vi "Load Drivers Dialog.vi"(8 "error in (no error)":errorcluster, 11 "Message Queue in":refnum<queue>) -> (0 "error out":errorcluster, 2 "Mssgs Sent":string, 5 "Asyncs":string[](array[string]), 7 "Syncs":string[](array[string]))   [LabVIEW 2014]
uses:
  APIs/Message Queue/Message Cluster.ctl
  APIs/Message Queue/Enqueue Message (Array).vi
  APIs/Message Queue/WINFAS 2 Message Queue.lvlib
panel:
  in  "LOAD":bool
  in  "Cancel":bool
  in  "Driver 5":path
  in  "Driver 4":path
  in  "Driver 3":path
  in  "Driver 2":path
  in  "Drivers Async":path[](array[path])=[path "", path "", path "", path "", path "", path "", path "", path "", path "", path ""]
  in  "Driver 1":path
  # "Drivers\nAsync"
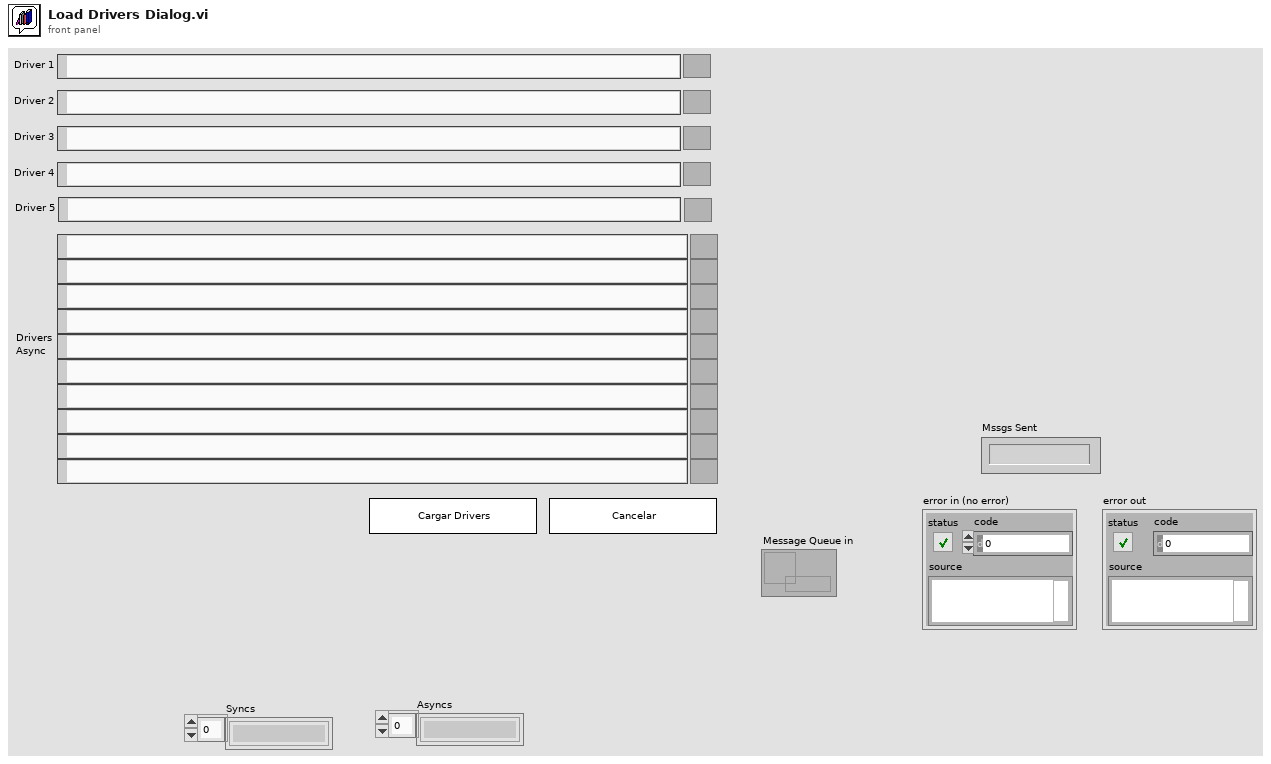
[diagram p1: front panel]
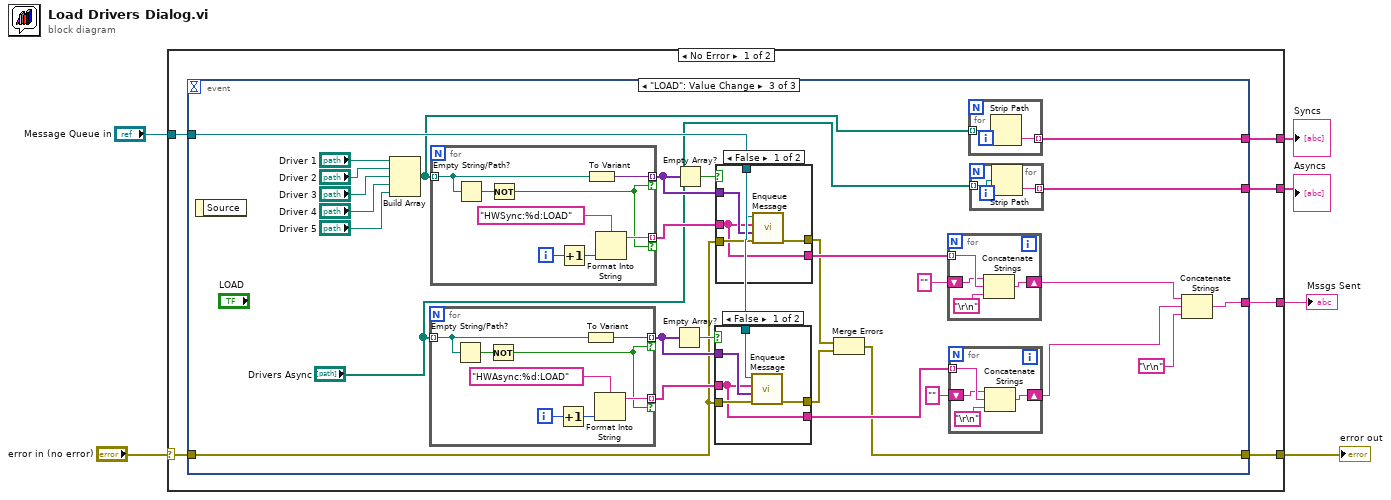
[diagram p0: block diagram]
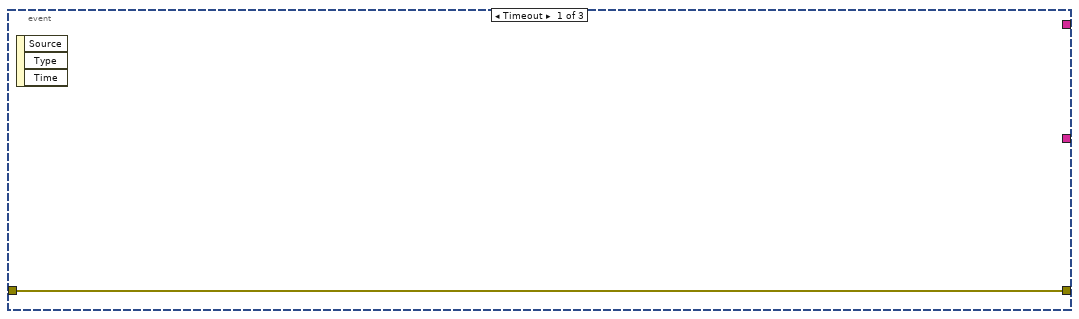
[diagram p2: hidden frame]
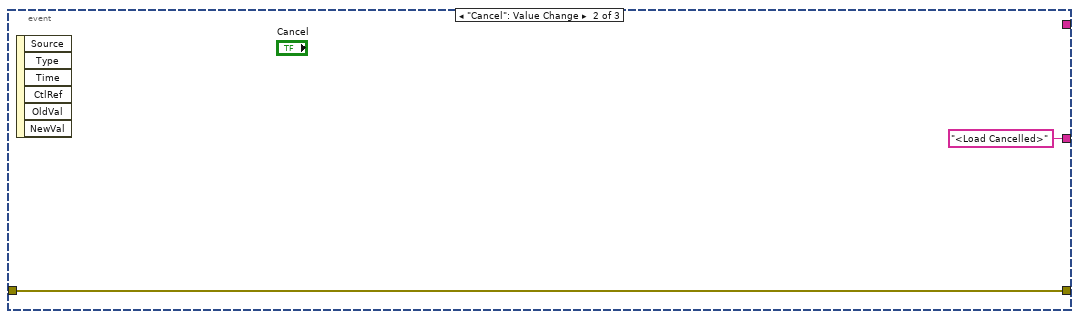
[diagram p3: hidden frame]
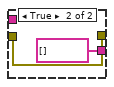
[diagram p4: hidden frame]
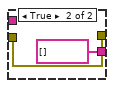
[diagram p5: hidden frame]
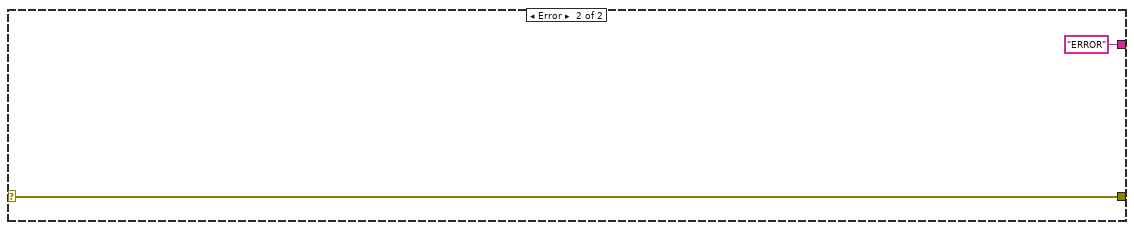
[diagram p6: hidden frame]
diagram:
  n1 = case shown="No Error" "error in (no error)" {
    selector: "error in (no error)" -> [w12 w87]
    tunnel: [w11 w87] -> w5
    tunnel: "Message Queue in" -> [w10 _]
    tunnel: [w9 "ERROR"] -> w3
    tunnel: [w8 _] -> w2
    tunnel: [w7 _] -> w1
    frame No Error {
      n2 = event shown="[2] \"LOAD\": Value Change" {
        selector: _ -> [_ _ _]
        dyn-events: _ -> [_ _ _]
        timeout: _ -> [_ _ _]
        tunnel: w12 -> [w13 w15 w20]
        tunnel: [w13 w15 w21] -> w11
        tunnel: w10 -> [_ _ w27]
        tunnel: [_ "<Load Cancelled>" w33] -> w9
        tunnel: [_ _ w17] -> w8
        tunnel: [_ _ w16] -> w7
        event Timeout {
          n3 = event-data() -> ()  [unwired: 1 in, 3 out]
        }
        event "Cancel": Value Change {
          n4 = event-data() -> ()  [unwired: 1 in, 6 out]
        }
        event "LOAD": Value Change {
          n5 = event-data() -> ()  [unwired: 1 in, 1 out]
          n6 = Build Array("Driver 1", "Driver 2", "Driver 3", "Driver 4", "Driver 5") -> (w19:path[])
          n7 = for {
            tunnel: "Drivers Async" -> [w62] mode=indexing
            tunnel: [w63] -> w29 mode=indexing if=w59
            tunnel: [w61] -> w30 mode=indexing if=w59
            i -> [w66]
            n8 = Empty String/Path?(string/path=w62) -> (empty?=w60:bool)
            n9 = Not(x=w60) -> (.not. x?=w59:bool)
            n10 = Increment(x=w66) -> (x+1=w64:i32)
            n11 = To Variant(anything=w62) -> (Variant=w61:variant)
            n12 = Format Into String(format string="HWAsync:%d:LOAD", w64) -> (resulting string=w63:string)  [unwired: 2 in, 1 out]
          }
          n13 = for {
            tunnel: w19 -> [w81] mode=indexing
            tunnel: [w82] -> w37 mode=indexing if=w78
            tunnel: [w80] -> w36 mode=indexing if=w78
            i -> [w85]
            n14 = Empty String/Path?(string/path=w81) -> (empty?=w79:bool)
            n15 = Not(x=w79) -> (.not. x?=w78:bool)
            n16 = Increment(x=w85) -> (x+1=w83:i32)
            n17 = To Variant(anything=w81) -> (Variant=w80:variant)
            n18 = Format Into String(format string="HWSync:%d:LOAD", w83) -> (resulting string=w82:string)  [unwired: 2 in, 1 out]
          }
          n19 = Empty Array?(array=w30) -> (empty?=w28:bool)
          n20 = Empty Array?(array=w36) -> (empty?=w38:bool)
          n21 = case shown="False" w28 {
            tunnel: [w56 w58] -> w22
            tunnel: w20 -> [w55 w58]
            tunnel: w27 -> [w54 _]
            tunnel: w29 -> [w52 _]
            tunnel: w30 -> [w53 _]
            tunnel: [w52 string[] []] -> w25
            frame False {
              n22 = call-poly "Enqueue Message.vi"("error in (no error)"=w55, "Message Data Array"=w53, "Message Array"=w52, "Message Queue"=w54) -> ("error out"=w56:errorcluster)  [unwired: 6 in, 1 out]
            }
            frame True {
            }
          }
          n23 = case shown="False" w38 {
            tunnel: [w75 w77] -> w23
            tunnel: w20 -> [w74 w77]
            tunnel: w27 -> [w73 _]
            tunnel: w37 -> [w71 _]
            tunnel: w36 -> [w72 _]
            tunnel: [w71 string[] []] -> w35
            frame False {
              n24 = call-poly "Enqueue Message.vi"("error in (no error)"=w74, "Message Data Array"=w72, "Message Array"=w71, "Message Queue"=w73) -> ("error out"=w75:errorcluster)  [unwired: 6 in, 1 out]
            }
            frame True {
            }
          }
          n25 = Merge Errors(w23, w22) -> (w21:errorcluster)
          n26 = for {
            tunnel: w35 -> [w70] mode=indexing
            shift-right: [w69] -> w34
            shift-left: "" -> [w68]
            n27 = Concatenate Strings(w68, w70, "\r\n") -> (w69:string)
          }
          n28 = for {
            tunnel: w25 -> [w51] mode=indexing
            shift-right: [w50] -> w24
            shift-left: "" -> [w49]
            n29 = Concatenate Strings(w49, w51, "\r\n") -> (w50:string)
          }
          n30 = for {
            tunnel: w19 -> [w47] mode=indexing
            tunnel: [w46] -> w17 mode=indexing
            n31 = Strip Path(path=w47) -> (name=w46:string)  [unwired: 1 out]
          }
          n32 = for {
            tunnel: "Drivers Async" -> [w45] mode=indexing
            tunnel: [w44] -> w16 mode=indexing
            n33 = Strip Path(path=w45) -> (name=w44:string)  [unwired: 1 out]
          }
          n34 = Concatenate Strings(w34, w24, "\r\n") -> (w33:string)
        }
      }
    }
    frame Error {
    }
  }
  "error out" <- w5
  "Mssgs Sent" <- w3
  "Syncs" <- w2
  "Asyncs" <- w1
